vi "(10) part 2 que.vi"() -> ()   [LabVIEW 2025]
panel:
  in  "operation (0:open) 4":T1(ring)
  out "error out 4":errorcluster
  in  "error in 4":errorcluster
  in  "Array 4":bool[](array[boolean])
  in  "operation (0:open) 3":T1(ring)
  out "error out 3":errorcluster
  in  "error in 3":errorcluster
  in  "Array 3":bool[](array[boolean])
  in  "operation (0:open) 2":T1(ring)
  out "error out 2":errorcluster
  in  "error in 2":errorcluster
  in  "Array 2":bool[](array[boolean])
  in  "operation (0:open)":T1(ring)
  out "error out":errorcluster
  in  "error in":errorcluster
  in  "Array":bool[](array[boolean])
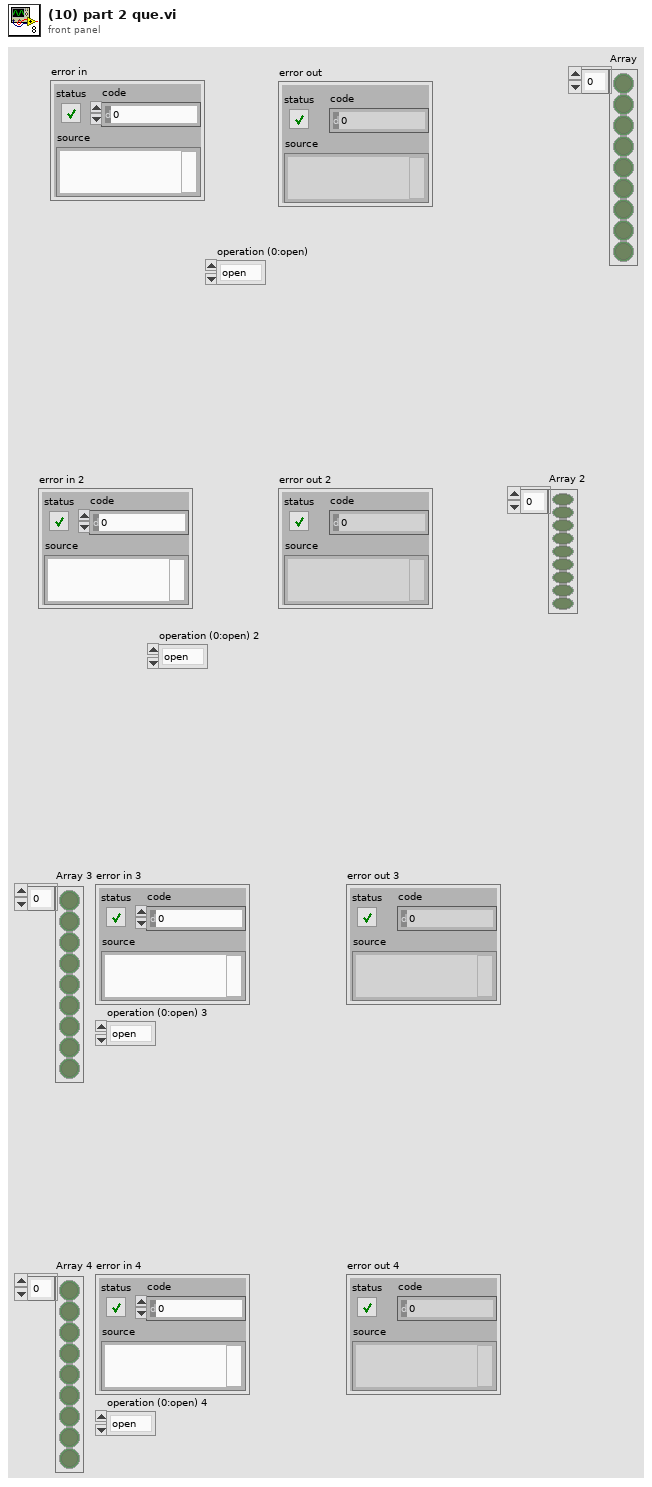
[diagram p1: front panel]
types:
  T1 = enum16{"open", "replace", "create", "open or create", "replace or create", "replace or create with confirmation"}
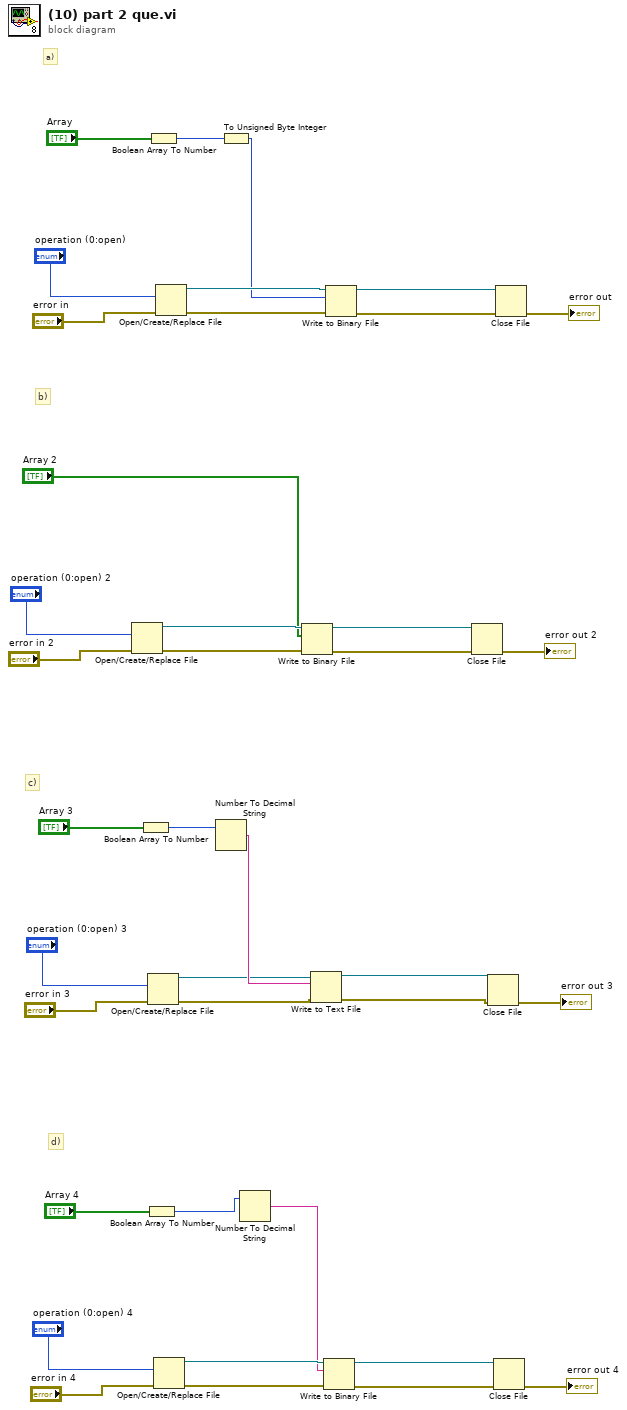
[diagram p0: block diagram]
diagram:
  # "d)"
  # "c)"
  # "b)"
  # "a)"
  n1 = Open/Create/Replace File(error in="error in 2", operation (0:open)="operation (0:open) 2") -> (refnum out=w25:refnum<file>, error out=w27:errorcluster)  [unwired: 4 in, 1 out]
  n2 = Boolean Array To Number(Boolean array="Array 3") -> (number=w16:u32)
  n3 = Boolean Array To Number(Boolean array="Array 4") -> (number=w1:u32)
  n4 = Open/Create/Replace File(error in="error in 3", operation (0:open)="operation (0:open) 3") -> (refnum out=w12:refnum<file>, error out=w15:errorcluster)  [unwired: 4 in, 1 out]
  n5 = Boolean Array To Number(Boolean array="Array") -> (number=w30:u32)
  n6 = Open/Create/Replace File(error in="error in 4", operation (0:open)="operation (0:open) 4") -> (refnum out=w7:refnum<file>, error out=w9:errorcluster)  [unwired: 4 in, 1 out]
  n7 = Open/Create/Replace File(error in="error in", operation (0:open)="operation (0:open)") -> (refnum out=w35:refnum<file>, error out=w37:errorcluster)  [unwired: 4 in, 1 out]
  n8 = Number To Decimal String(number=w16) -> (decimal integer string=w13:string)  [unwired: 1 in]
  n9 = To Unsigned Byte Integer(number=w30) -> (unsigned 8bit integer=w29:u8)
  n10 = Number To Decimal String(number=w1) -> (decimal integer string=w2:string)  [unwired: 1 in]
  n11 = Write to Binary File(file (use dialog)=w25, data="Array 2", error in=w27) -> (refnum out=w24:refnum<file>, error out=w26:errorcluster)  [unwired: 3 in, 1 out]
  n12 = Write to Text File(file (use dialog)=w12, text=w13, error in=w15) -> (refnum out=w11:refnum<file>, error out=w14:errorcluster)  [unwired: 1 in, 1 out]
  n13 = Write to Binary File(file (use dialog)=w7, data=w2, error in=w9) -> (refnum out=w6:refnum<file>, error out=w8:errorcluster)  [unwired: 3 in, 1 out]
  n14 = Write to Binary File(file (use dialog)=w35, data=w29, error in=w37) -> (refnum out=w34:refnum<file>, error out=w36:errorcluster)  [unwired: 3 in, 1 out]
  n15 = Close File(refnum=w24, error in=w26) -> (error out=→"error out 2":errorcluster)  [unwired: 1 out]
  n16 = Close File(refnum=w11, error in=w14) -> (error out=→"error out 3":errorcluster)  [unwired: 1 out]
  n17 = Close File(refnum=w6, error in=w8) -> (error out=→"error out 4":errorcluster)  [unwired: 1 out]
  n18 = Close File(refnum=w34, error in=w36) -> (error out=→"error out":errorcluster)  [unwired: 1 out]
